vi "shim_heater_init.vi"(8 "error in":errorcluster, 10 "port":u16=6722, 11 "address":string="192.168.24.184") -> (0 "error out":errorcluster, 1 "ch2":bool, 2 "ch1":bool, 3 "conn_id":refnum<k5>, 4 "status":bool, 6 "message":string)   [LabVIEW 2019]
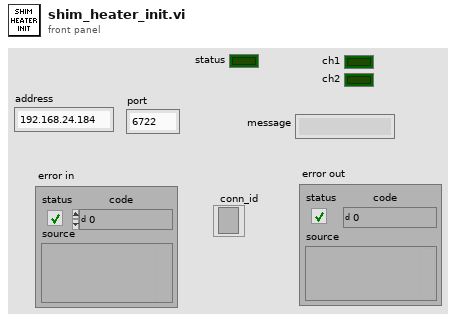
[diagram p1: front panel]
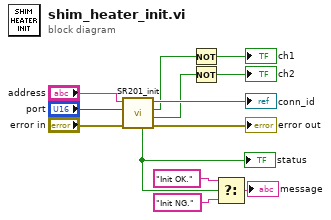
[diagram p0: block diagram]
diagram:
  n1 = call "SR201_init.vi"("error in"="error in", "port"="port", "address"="address") -> ("error out"=→"error out":errorcluster, "ch2"=w10:bool, "ch1"=w6:bool, "conn_id"=→"conn_id":refnum<k5>, "status"=w1:bool)  [unwired: 4 in]
  "status" <- w1
  n2 = Not(x=w6) -> (.not. x?=→"ch1":bool)
  n3 = Not(x=w10) -> (.not. x?=→"ch2":bool)
  n4 = Select(t="Init OK." ("message"), s=w1, f="Init NG." ("message")) -> (s? t:f=→"message":string)
